vi "p2.6.vi"() -> ()   [LabVIEW 2020]
panel:
  in  "Pos Vertical":dbl(slide) scale=0.0..10.0
  in  "Frecuencia (Hz)":dbl(knob) scale=0.0..10.0
  in  "stop":bool
  out "error out":errorcluster
  out "Canal dcho":dbl[](graph)
  out "Canal izqdo":dbl[](graph)
  in  "fs DA (Hz)":dbl=-1.0
  in  "fs AD (Hz)":dbl=40000.0
  in  "device name":tag="myDAQ1"
  in  "Num muestras":i32
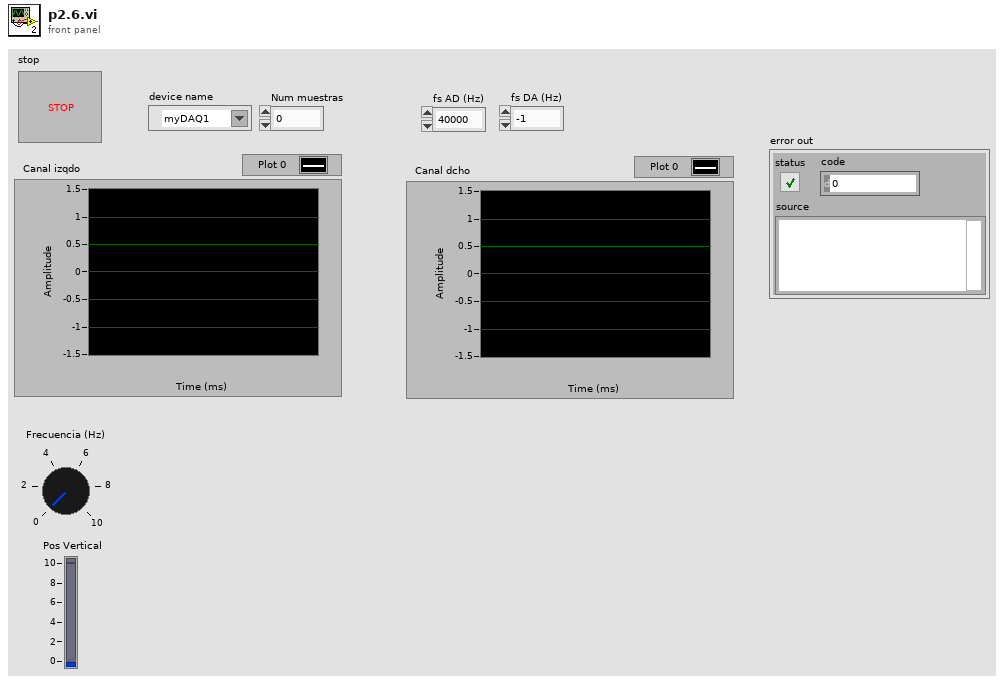
[diagram p1: front panel]
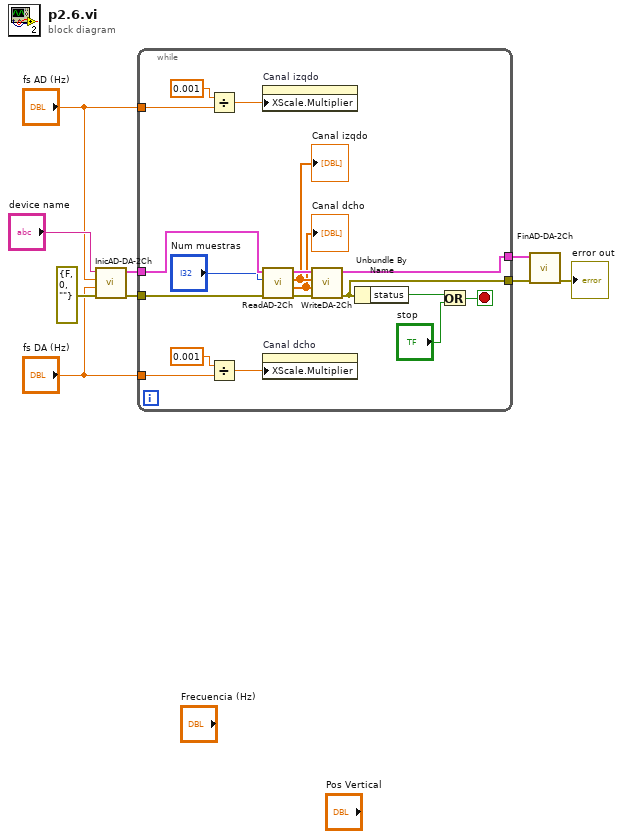
[diagram p0: block diagram]
diagram:
  n1 = call <userlib>:"InicAD-DA-2Ch.vi"("error in"=errorcluster {"status"=FALSE, "code"=0, "source"=""}, "fs DA (Hz)"="fs DA (Hz)", "fs AD (Hz)"="fs AD (Hz)", "device name"="device name") -> ("error out"=w8:errorcluster, "Tarea Out"=w9:cluster{"AD":refnum<k21>, "DA":refnum<k21>})  [unwired: 6 in]
  n2 = while {
    tunnel: w9 -> [w27]
    tunnel: w8 -> [w26]
    tunnel: [w18] -> w7
    tunnel: [w23] -> w6
    tunnel: "fs AD (Hz)" -> [w16]
    tunnel: "fs DA (Hz)" -> [w15]
    stop <- w19 stop-if-true
    n3 = Divide(x=0.001, y=w16) -> (x/y=w12:dbl)
    n4 = Divide(x=0.001, y=w15) -> (x/y=w11:dbl)
    n5 = property on="Canal izqdo" class="WFGraph (strict)"("XScale.Multiplier"=w12) -> ()  [unwired: 2 in, 2 out]
    n6 = call <userlib>:"ReadAD-2Ch.vi"("error in"=w26, "numero de muestras"="Num muestras", "Tarea In"=w27) -> ("error out"=w25:errorcluster, "Data Right"=w20:dbl[], "Data Left"=w21:dbl[], "Tarea Out"=w24:cluster{"AD":refnum<k21>, "DA":refnum<k21>})  [unwired: 5 in]
    "Canal izqdo" <- w21
    "Canal dcho" <- w20
    n7 = property on="Canal dcho" class="WFGraph (strict)"("XScale.Multiplier"=w11) -> ()  [unwired: 2 in, 2 out]
    n8 = call <userlib>:"WriteDA-2Ch.vi"("error in"=w25, "Data Right"=w20, "Data Left"=w21, "Tarea In"=w24) -> ("error out"=w18:errorcluster, "Tarea Out"=w23:cluster{"AD":refnum<k21>, "DA":refnum<k21>})  [unwired: 6 in]
    n9 = Unbundle By Name(w18) -> ("status"=w17:bool)
    n10 = Or(x=w17, y="stop") -> (x .or. y?=w19:bool)
  }
  n11 = call <userlib>:"FinAD-DA-2Ch.vi"("error in"=w7, "Tarea In"=w6) -> ("error out"=→"error out":errorcluster)  [unwired: 9 in]
